vi "InsertExactRows.vi"(6 "# rows":i32, 7 "Table History ref":refnum<vi>, 8 "error in (no error)":errorcluster, 9 "Table CtlRef In":refnum<vi>, 10 "Row":i32, 11 "Col Array Ref in":refnum<vi>) -> (0 "error out":errorcluster, 1 "Table CtlRef Out":refnum<vi>, 3 "Col Array Ref out":refnum<vi>)   [LabVIEW 2013]
doc: "Inserts \"# rows\" copies of \"Row\" after Row, copying formatting, and re-numbering rows; also updates Table History (if Table History ref is wired)."
uses:
  TypeDefs/TableHistory.ctl
  TypeDefs/TableArray.ctl
  <vilib>/Utility/miscctls.llb/LVRowAndColumnTypeDef.ctl
  ColumnVIs/Column/Column.lvclass
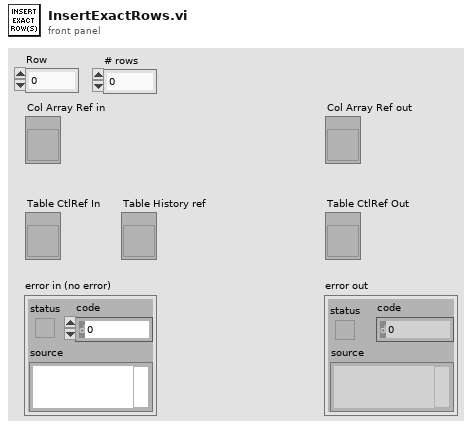
[diagram p1: front panel]
types:
  T1 = typedef "LVRowAndColumnTypeDef.ctl" = cluster{"Row":i32, "Column":i32}
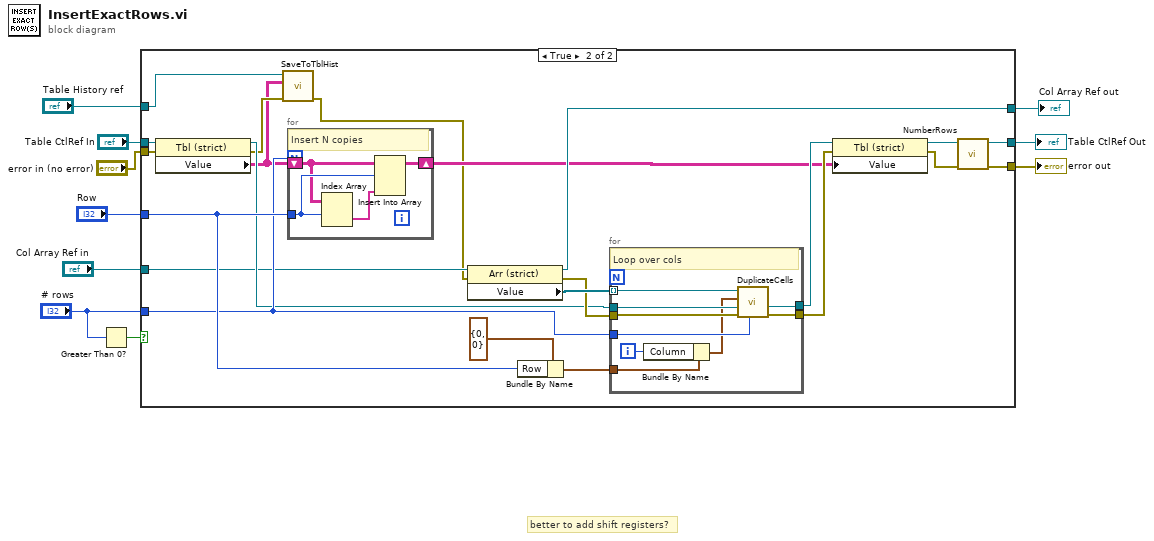
[diagram p0: block diagram]
diagram:
  # "better to add shift registers?"
  n1 = Greater Than 0?(x="# rows") -> (x > 0?=w4:bool)
  n2 = case shown="True" w4 {
    tunnel: "Table CtlRef In" -> [w13 w35]
    tunnel: "error in (no error)" -> [w12 w34]
    tunnel: [w12 w15] -> w8
    tunnel: [w13 w14] -> w7
    tunnel: "Row" -> [_ w29]
    tunnel: [w11 w26] -> w5
    tunnel: "# rows" -> [_ w25]
    tunnel: "Col Array Ref in" -> [w11 w22]
    tunnel: "Table History ref" -> [_ w18]
    frame False {
    }
    frame True {
      n3 = property class="Tbl (strict)"(reference=w35, error in=w34) -> (reference out=w23:refnum<vi>, error out=w21:errorcluster, "Value"=w19:string[][])
      n4 = call "SaveToTblHist.vi"("error in (no error)"=w21, "OldTable (reset)"=w19, "Table History ref"=w18) -> ("error out"=w20:errorcluster)  [unwired: 8 in]
      n5 = for {
        N: w25 -> [_]
        tunnel: w29 -> [w39]
        shift-right: [w36] -> w24
        shift-left: w19 -> [w38]
        # "Insert N copies"
        n6 = Index Array(array=w38, index (row)=w39) -> (element=w37:string[])  [unwired: 1 in]
        n7 = Insert Into Array(array=w38, index (row)=w39, new element=w37) -> (w36:string[][])  [unwired: 1 in]
      }
      n8 = property class="Arr (strict)"(reference=w22, error in=w20) -> (reference out=w26:refnum<vi>, error out=w32:errorcluster, "Value"=w33:refnum<class "Column.lvclass">[])
      n9 = Bundle By Name(cluster=T1 {"Row"=0, "Column"=0} ("Active Cell:Active Cell"), "Row"=w29) -> (w30:T1)
      n10 = for {
        tunnel: w23 -> [w46]
        tunnel: w32 -> [w47]
        tunnel: [w45] -> w28
        tunnel: [w44] -> w27
        tunnel: w33 -> [w43] mode=indexing
        tunnel: w25 -> [w42]
        tunnel: w30 -> [w41]
        i -> [w48]
        # "Loop over cols"
        n11 = Bundle By Name(cluster=w41, "Column"=w48) -> (w40:T1)
        n12 = call-dynamic "DuplicateCells.vi"("# Rows"=w42, "error in (no error)"=w47, "Table CtlRef In"=w46, "Cell Position"=w40, "Column in"=w43) -> ("error out"=w44:errorcluster, "Table CtlRef Out"=w45:refnum<vi>)  [unwired: 4 in, 1 out]
      }
      n13 = property class="Tbl (strict)"(reference=w28, error in=w27, "Value"=w24) -> (reference out=w17:refnum<vi>, error out=w16:errorcluster)
      n14 = call "NumberRows.vi"("error in (no error)"=w16, "Table Ref in"=w17) -> ("error out"=w15:errorcluster, "Table Ref out"=w14:refnum<vi>)  [unwired: 8 in]
    }
  }
  "error out" <- w8
  "Table CtlRef Out" <- w7
  "Col Array Ref out" <- w5
